vi "Test Numeric Measured Value Properly Formatted for Small numbers.vi"(11 "Test Case In":refnum<class "Report CSV Content Test.lvclass">) -> (0 "error out":errorcluster, 3 "Test Case Out":refnum<class "Report CSV Content Test.lvclass">)   [LabVIEW 2020, in "Report CSV Content Test.lvclass"]
uses:
  Report CSV Content Test.lvclass
  Report CSV Content Test.lvclass/Report CSV Content Test.ctl
  source/Test Result Handler/TestStand Result Handler.lvclass
  Mock Configuration/Mock Configuration.lvclass
  <vilib>/Astemes/LUnit/Palette/Advanced Assertions/LUnit Advanced Assertions.lvlib
  C:/git/danfoss-csv-report-teststand-plugin/source/Configuration/Configuration.lvclass
  C:/Program Files (x86)/National Instruments/LabVIEW 2020/vi.lib/Astemes/LUnit/Test Case.lvclass
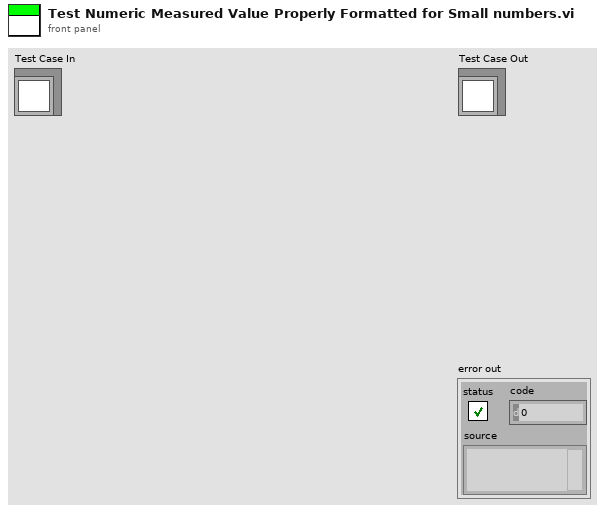
[diagram p1: front panel]
types:
  T1 = typedef "Astemes_CSVReportPlugin.lvlib/TestStand Result Handler.lvclass/TestStand Result.ctl" = cluster{"error in (no error)":errorcluster, "ReportText":string, "TS":cluster{"Index":i32, "BlockLevel":i32, "StartTime":dbl, "Id":i32, "StepType":string, "StepID":string, "StepGroup":string, "StepName":string}, "Status":string}
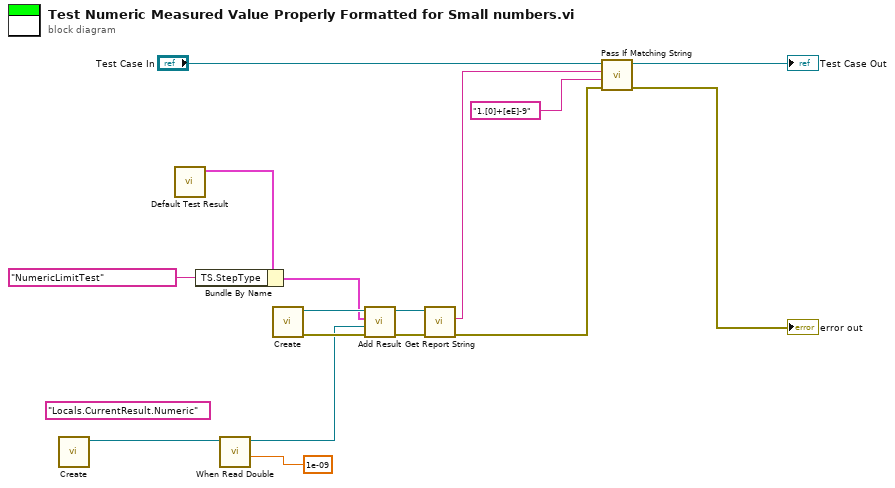
[diagram p0: block diagram]
diagram:
  (unwired) "Locals.CurrentResult.Numeric" ("key")
  n1 = call "Create.vi"() -> ("Mock Class Generator out"=w11:refnum<class "Mock Configuration.lvclass">)  [unwired: 10 in, 1 out]
  n2 = call "Default Test Result.vi"() -> ("TestStand Result"=w14:T1)  [unwired: 11 in]
  n3 = Bundle By Name(cluster=w14, "TS.StepType"="NumericLimitTest" ("Status")) -> (w13:T1)
  n4 = call "When Read Double.vi"("value"=1e-09, "Configuration In"=w11) -> ("Configuration Out"=w10:refnum<class "Mock Configuration.lvclass">)  [unwired: 9 in]
  n5 = call "Create.vi"() -> ("error out"=w15:errorcluster, "Test Result Handler"=w16:refnum<class "TestStand Result Handler.lvclass">)  [unwired: 10 in]
  n6 = call "Add Result.vi"("error in (no error)"=w15, "Sequenc Context"=w10, "TestStand Result"=w13, "TestStand Result Handler In"=w16) -> ("error out"=w8:errorcluster, "TestStand Result Handler Out"=w9:refnum<class "TestStand Result Handler.lvclass">)  [unwired: 6 in]
  n7 = call "Get Report String.vi"("error in (no error)"=w8, "TestStand Result Handler In"=w9) -> ("error out"=w7:errorcluster, "Report Text"=w2:string)  [unwired: 8 in]
  n8 = call <vilib>:"Pass If Matching String.vi"("error in (no error)"=w7, "Regular Expression"="1.[0]+[eE]-9" ("Report Text"), "String"=w2, "LUnit Test Case In"="Test Case In") -> ("error out"=→"error out":errorcluster, "LUnit Test Case Out"=→"Test Case Out":refnum<class "Report CSV Content Test.lvclass">)  [unwired: 6 in]
